vi "DB_查询通讯设备名称列表.vi"(8 "error in (no error)":errorcluster caption="错误输入（无错误）") -> (0 "error out":errorcluster caption="错误输出", 3 "通讯设备列表名":string[](array[string]))   [LabVIEW 2018]
uses:
  <vilib>/drjdpowell/SQLite Library/SQL Connection/Connection.lvclass
  <vilib>/drjdpowell/SQLite Library/SQL Connection/Open (path).vi
  <vilib>/JDP Science/JDP Science Common Utilities/Trim Whitespace__JDP.vi
  <vilib>/drjdpowell/SQLite Library/SQL Connection/Open (string).vi
  <vilib>/AdvancedString/Path To Command Line String.vi
  <vilib>/drjdpowell/SQLite Library/SQL Connection/Execute SQL (1D String).vi
  <vilib>/drjdpowell/SQLite Library/SQLite.lvlib
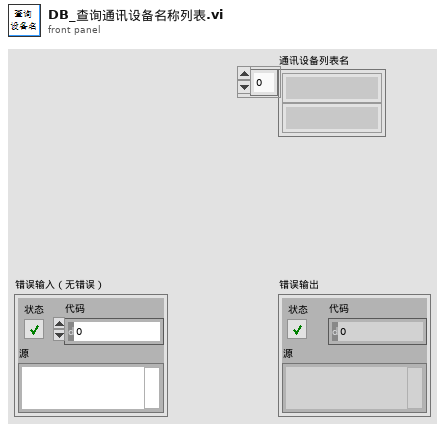
[diagram p1: front panel]
types:
  T1 = enum16{"New or existing", "Existing", "Read only"}
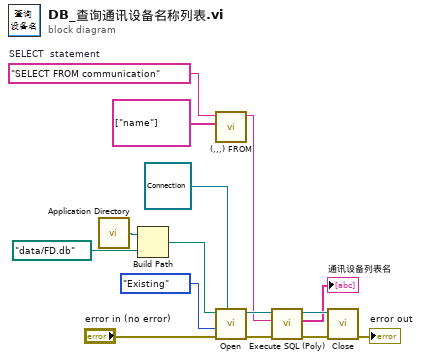
[diagram p0: block diagram]
diagram:
  w6 = "SELECT FROM communication"  # SELECT  statement
  n1 = call <vilib>:"Application Directory.vi"() -> ("Application Directory"=w15:path)
  n2 = Build Path(base path=w15, name or relative path=path "data/FD.db" ("Application Directory")) -> (appended path=w13:path)
  n3 = call <vilib>:"(,,,) FROM.vi"("Column Names"=string[] ["name"] ("列首字符串[]"), "SQL containing FROM clause"=w6) -> ("SQL"=w4:string)  [unwired: 9 in]
  n4 = call-poly <vilib>:"Open.vi"("SQLite Connection type"=refnum<class "Connection.lvclass"> refnum, "error in (no error)"="error in (no error)", "File Option"=T1."Existing", "db file"=w13) -> ("error out"=w8:errorcluster, "SQLite Connection"=w10:refnum<class "Connection.lvclass">)  [unwired: 6 in]
  n5 = call-poly <vilib>:"Execute SQL (Poly).vi"("error in (no error)"=w8, "SQL"=w4, "SQLite Connection in"=w10) -> ("error out"=w7:errorcluster, "Result Set"=→"通讯设备列表名":string[], "SQLite Connection"=w9:refnum<class "Connection.lvclass">)  [unwired: 5 in, 1 out]
  n6 = call-dynamic "Close.vi"("error in (no error)"=w7, "SQLite Connection in"=w9) -> ("error out"=→"error out":errorcluster)  [unwired: 9 in]
